vi "WhileLoop.vi"() -> ()   [LabVIEW 2020]
panel:
  in  "milliseconds to wait":u32
  in  "stop":bool
  out "Tank":dbl(slide) scale=0.0..10.0
  in  "Slide":dbl(slide) scale=0.0..10.0
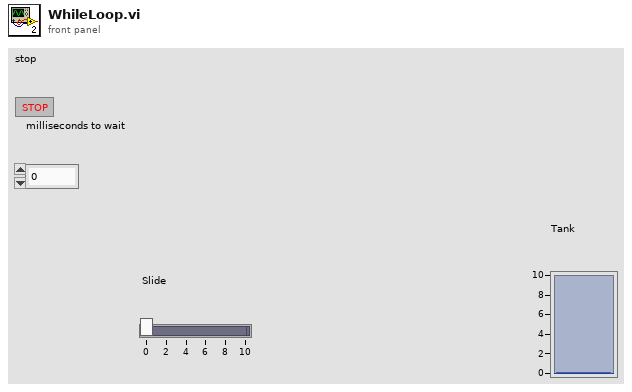
[diagram p1: front panel]
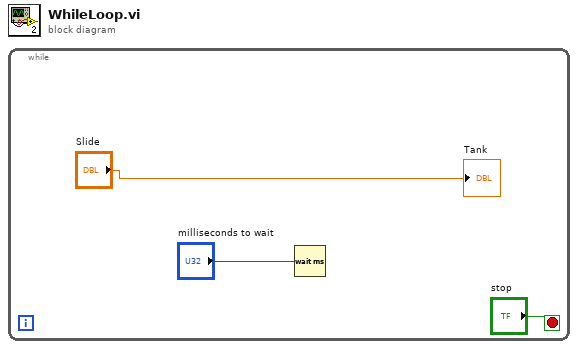
[diagram p0: block diagram]
diagram:
  n1 = while {
    stop <- "stop" stop-if-true
    n2 = Wait (ms)(milliseconds to wait="milliseconds to wait") -> ()  [unwired: 1 out]
    "Tank" <- "Slide"
  }
